vi "SysInfo-Get LabVIEW Version.vi"() -> (8 "Version Info":string)   [LabVIEW 2020]
uses:
  <resource>/objmgr/daqmx.rc
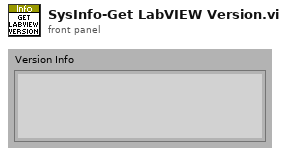
[diagram p1: front panel]
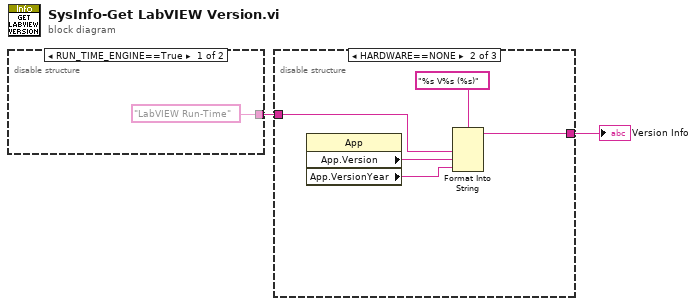
[diagram p0: block diagram]
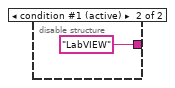
[diagram p2: hidden frame]
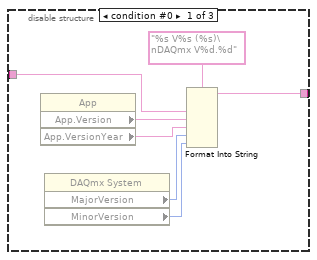
[diagram p3: hidden frame]
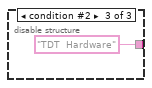
[diagram p4: hidden frame]
diagram:
  n1 = disable-structure shown="RUN_TIME_ENGINE==True" {
    disable-tunnel: ["LabVIEW Run-Time" "LabVIEW"] -> w1
    frame condition #0 {
    }
    frame condition #1 (active) {
    }
  }
  n2 = disable-structure shown="HARDWARE==NONE" {
    disable-tunnel: [w8 w13 "TDT  Hardware" ("string")] -> w2
    disable-tunnel: w1 -> [w5 w12 _]
    frame condition #0 {
      n3 = property class="App"() -> ("App.Version"=w10:string, "App.VersionYear"=w9:string)  [unwired: 2 in, 2 out]
      n4 = property class="DAQmx System"() -> ("MajorVersion"=w7:u32, "MinorVersion"=w6:u32)  [unwired: 2 in, 2 out]
      n5 = Format Into String(format string="%s V%s (%s)\nDAQmx V%d.%d", w5, w10, w9, w7, w6) -> (resulting string=w8:string)  [unwired: 2 in, 1 out]
    }
    frame condition #1 (active) {
      n6 = property class="App"() -> ("App.Version"=w15:string, "App.VersionYear"=w14:string)  [unwired: 2 in, 2 out]
      n7 = Format Into String(format string="%s V%s (%s)", w12, w15, w14) -> (resulting string=w13:string)  [unwired: 2 in, 1 out]
    }
    frame condition #2 {
    }
  }
  "Version Info" <- w2
